vi "del.vi"() -> ()   [LabVIEW 2025]
uses:
  Table_Filtering/Table_Filtering.lvlib
panel:
  in  "Sort Type":enum16{"numerical", "hex", "string"}(ring)
  in  "Sort by":u16(ring) items=["Packet_Number", "Timestamp", "Source", "Destination", "Protocol", "Length", "Data"]
  in  "Unsorted Data":string[][](array[string])=array1500x7[10500 elements]
  out "Table Control":string[][](table)
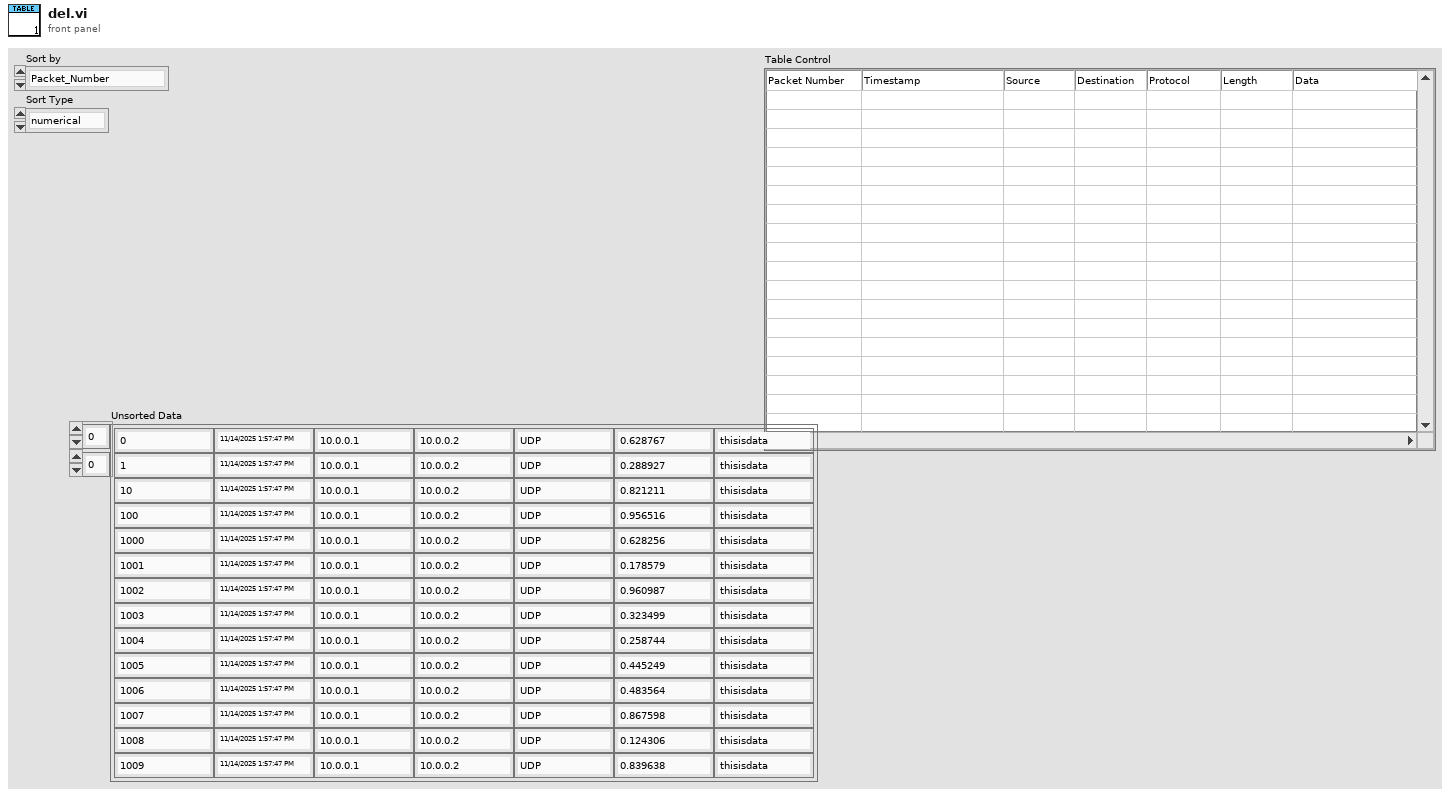
[diagram p1: front panel]
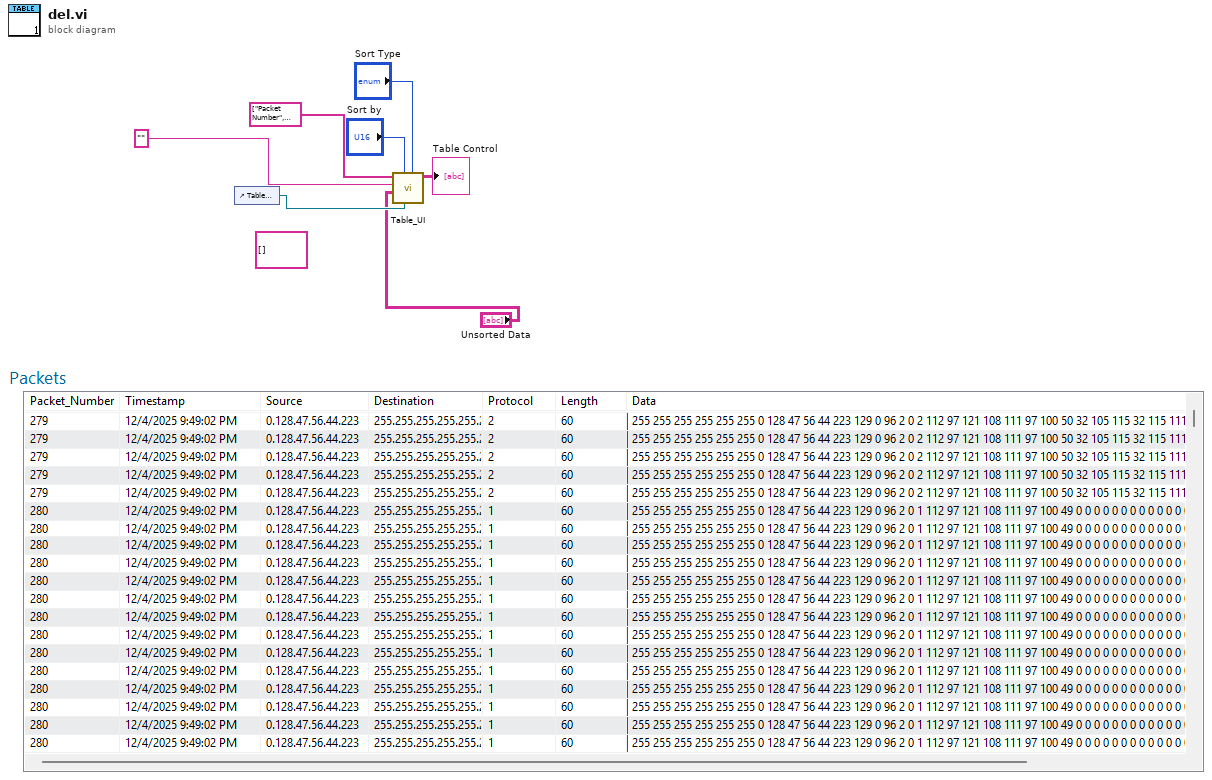
[diagram p0: block diagram]
diagram:
  (unwired) string[][] [] ("Table Control")
  n1 = control-ref of="Table Control"() -> (w6:refnum<vi>)
  n2 = call "Table_UI.vi"("Sort Type"="Sort Type", "Table Control Reference"=w6, "Sort by"="Sort by", "Prefiltered Data"="Unsorted Data", "Filter String"="", "Headers"=string[] ["Packet Number", "Timestamp", "Source", "Destination", "Protocol", "Length", "Data"]) -> ("Table Control"=→"Table Control":string[][])  [unwired: 4 in, 1 out]
